vi "String to Float.vi"(1 "string":string) -> (0 "float":dbl)   [LabVIEW 2017, in "Drivers.lvlib" / "ASI TG-1000.lvlib"]
uses:
  ASI TG-1000.lvlib
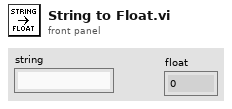
[diagram p1: front panel]
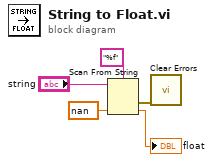
[diagram p0: block diagram]
diagram:
  n1 = Scan From String(format string="%f", input string="string", default 1=nan ("default value 1")) -> (error out=w2:errorcluster, output 1=→"float":dbl)  [unwired: 2 in, 2 out]
  n2 = call <vilib>:"Clear Errors.vi"("error in (no error)"=w2) -> ()  [unwired: 5 in, 2 out]
